vi "F5xxx_set_pulse_timing.vi"(8 "error in":errorcluster, 9 "pulse period":dbl, 10 "pulse width":dbl, 11 "VISA in":refnum<visa-resource-name>) -> (0 "error out":errorcluster, 3 "VISA out":refnum<visa-resource-name>)   [LabVIEW 2013]
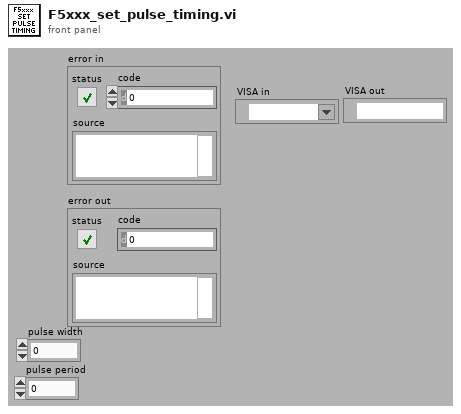
[diagram p1: front panel]
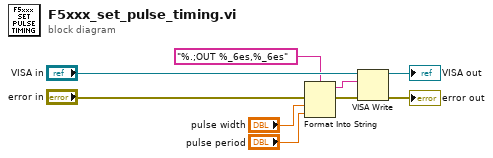
[diagram p0: block diagram]
diagram:
  n1 = Format Into String(format string="%.;OUT %_6es,%_6es", error in="error in", "pulse width", "pulse period") -> (resulting string=w4:string, error out=w6:errorcluster)  [unwired: 1 in]
  n2 = VISA Write(VISA resource name="VISA in", write buffer=w4, error in (no error)=w6) -> (VISA resource name out=→"VISA out":refnum<visa-resource-name>, error out=→"error out":errorcluster)  [unwired: 1 out]
